vi "Get Valid Channels to Update.vi"(8 "error in (no error)":errorcluster, 10 "Data Read":cluster{waveform(dbl)[], string[]}, 11 "Plugin in":refnum<class "StreamReader.lvclass">) -> (0 "error out":errorcluster, 2 "Waveforms Out":waveform(dbl)[](array[waveform]), 3 "Channels Out":string[](array[string]))   [LabVIEW 2024, in "StreamReader.lvlib" / "StreamReader.lvclass"]
uses:
  StreamReader.lvclass
  C:/Program Files/National Instruments/LabVIEW 2024/vi.lib/FlexLogger/SDK/PluginSDK.lvlibp/PEFClasses/SDK/Plugin/Plugin.lvclass
  <vilib>/FlexLogger/SDK/PluginSDK.lvlibp/PEFClasses/SDK/Producer Channel/Producer Channel.lvclass
  C:/Program Files/National Instruments/LabVIEW 2024/vi.lib/FlexLogger/SDK/PluginSDK.lvlibp/PEFClasses/SDK/Channel/Channel.lvclass
  <vilib>/FlexLogger/SDK/PluginSDK.lvlibp/PEFClasses/SDK/Plugin/Read Channels.vi
  <vilib>/FlexLogger/SDK/PluginSDK.lvlibp/PEFClasses/SDK/Plugin/Get Valid Producer Channels.vi
  <vilib>/FlexLogger/SDK/PluginSDK.lvlibp/PEFClasses/SDK/Channel/Channel.lvclass
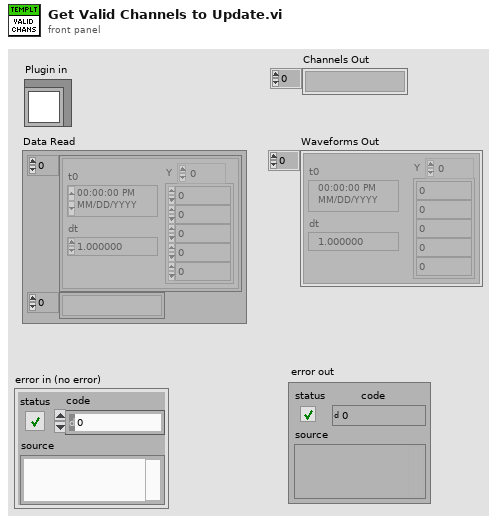
[diagram p1: front panel]
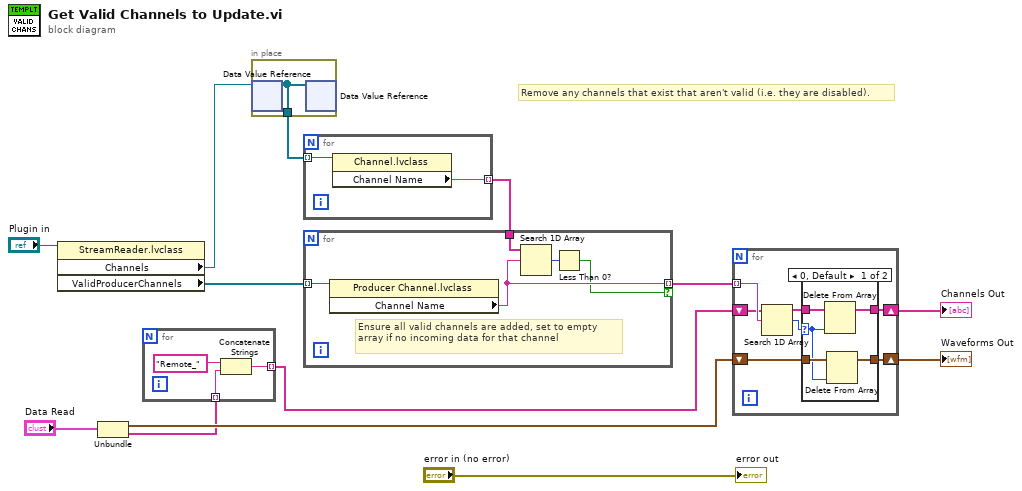
[diagram p0: block diagram]
diagram:
  # "Remove any channels that exist that aren't valid (i.e. they are disabled)."
  n1 = property class="StreamReader.lvclass"(reference="Plugin in") -> ("Channels"=w9:refnum<data-value>, "ValidProducerChannels"=w11:refnum<class "Producer Channel.lvclass">[])  [unwired: 1 in, 2 out]
  n2 = Unbundle("Data Read") -> (w7:waveform(dbl)[], w3:string[])
  n3 = for {
    tunnel: w3 -> [w15] mode=indexing
    tunnel: [w14] -> w6 mode=indexing
    n4 = Concatenate Strings("Remote_" ("string"), w15) -> (w14:string)
  }
  n5 = in-place {
    in-place-border: [w17] -> w8
    n6 = in-place-dvr #1(w9) -> (w17:refnum<class "Channel.lvclass">[])  [unwired: 1 out]
    n7 = in-place-dvr #1(w17) -> ()  [unwired: 2 out]
  }
  n8 = for {
    tunnel: w8 -> [w19] mode=indexing
    tunnel: [w18] -> w2 mode=indexing
    n9 = property class="Channel.lvclass"(reference=w19) -> ("Channel Name"=w18:string)  [unwired: 1 in, 2 out]
  }
  n10 = for {
    tunnel: w11 -> [w24] mode=indexing
    tunnel: w2 -> [w23]
    tunnel: [w22] -> w1 mode=indexing if=w20
    # "Ensure all valid channels are added, set to empty array if no incoming data for that channel"
    n11 = property class="Producer Channel.lvclass"(reference=w24) -> ("Channel Name"=w22:string)  [unwired: 1 in, 2 out]
    n12 = Search 1D Array(1D array=w23, element=w22) -> (index of element=w21:i32)  [unwired: 1 in]
    n13 = Less Than 0?(x=w21) -> (x < 0?=w20:bool)
  }
  n14 = for {
    shift-right: [w25] -> w5
    shift-left: w7 -> [w27]
    shift-right: [w26] -> w4
    shift-left: w6 -> [w28]
    tunnel: w1 -> [w30] mode=indexing
    n15 = Search 1D Array(1D array=w28, element=w30) -> (index of element=w29:i32)  [unwired: 1 in]
    n16 = case shown="0, Default" w29 {
      selector: w29 -> [w33 _]
      tunnel: w28 -> [w34 w37]
      tunnel: w27 -> [w35 w36]
      tunnel: [w32 w37] -> w26
      tunnel: [w31 w36] -> w25
      frame 0, Default {
        n17 = Delete From Array(array=w34, index=w33) -> (array with subset deleted=w32:string[])  [unwired: 1 in, 1 out]
        n18 = Delete From Array(array=w35, index=w33) -> (array with subset deleted=w31:waveform(dbl)[])  [unwired: 1 in, 1 out]
      }
      frame -1 {
      }
    }
  }
  "Channels Out" <- w4
  "Waveforms Out" <- w5
  "error out" <- "error in (no error)"
